vi "MS_on_off_sorting.vi"(4 "Laser gate threshold":dbl, 5 "gate_trace":waveform(dbl), 6 "Number of sweeps":i32, 7 "data_trace":waveform(dbl), 8 "IR_on_q_error_in":errorcluster, 9 "IR_on_q_in":refnum<queue>, 10 "IR_off_q_error_in":errorcluster, 11 "IR_off_q_in":refnum<queue>) -> (0 "IR_on_q_error_out":errorcluster, 1 "IR_on_q_out":refnum<queue>, 2 "IR_off_q_error_out":errorcluster, 3 "IR_off_q_out":refnum<queue>)   [LabVIEW 2020]
uses:
  <vilib>/Waveform/WDTOps.llb/WDT Number of Waveform Samples DBL.vi
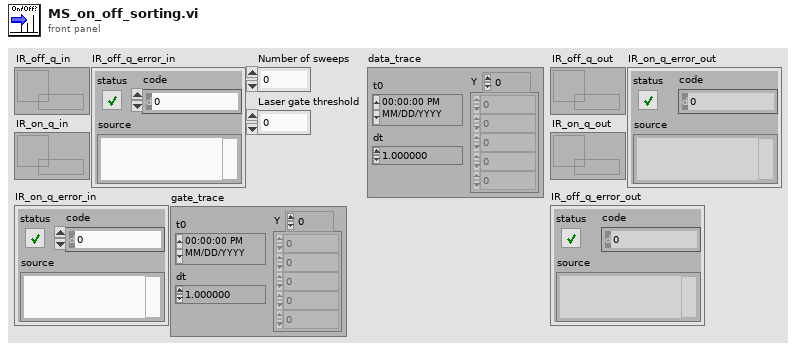
[diagram p1: front panel]
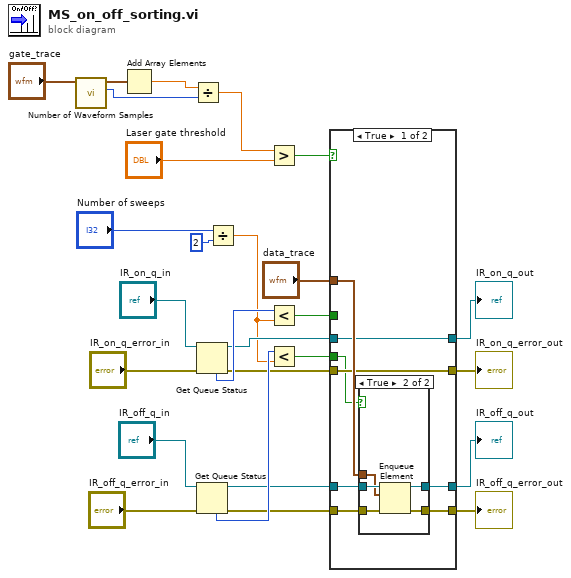
[diagram p0: block diagram]
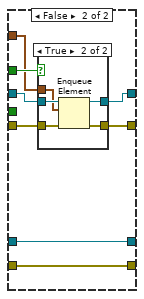
[diagram p3: hidden frame]
diagram:
  n1 = call-poly <vilib>:"Number of Waveform Samples.vi"("waveform in"="gate_trace") -> ("number of samples"=w13:i32, "waveform out"=w15:waveform(dbl))  [unwired: 8 in, 1 out]
  n2 = Add Array Elements(numeric array=w15) -> (sum=w14:dbl)
  n3 = Divide(x=w14, y=w13) -> (x/y=w18:dbl)
  n4 = Get Queue Status(queue="IR_on_q_in", error in (no error)="IR_on_q_error_in") -> (queue out=w10:refnum<queue>, error out=w9:errorcluster, # elements in queue=w20:i32)  [unwired: 1 in, 5 out]
  n5 = Get Queue Status(queue="IR_off_q_in", error in (no error)="IR_off_q_error_in") -> (queue out=w12:refnum<queue>, error out=w11:errorcluster, # elements in queue=w21:i32)  [unwired: 1 in, 5 out]
  n6 = Divide(x="Number of sweeps", y=2) -> (x/y=w2:dbl)
  n7 = Greater?(x=w18, y="Laser gate threshold") -> (0:w19:bool)
  n8 = Less?(x=w20, y=w2) -> (x < y?=w1:bool)
  n9 = Less?(x=w21, y=w2) -> (x < y?=w3:bool)
  n10 = case shown="True" w19 {
    tunnel: w12 -> [w35 w46]
    tunnel: w11 -> [w34 w45]
    tunnel: w10 -> [w30 w49]
    tunnel: w9 -> [w29 w48]
    tunnel: w1 -> [_ w50]
    tunnel: "data_trace" -> [w33 w47]
    tunnel: [w32 w46] -> w7
    tunnel: [w31 w45] -> w4
    tunnel: [w30 w44] -> w6
    tunnel: [w29 w43] -> w5
    tunnel: w3 -> [w28 _]
    frame True {
      n11 = case shown="True" w28 {
        tunnel: w35 -> [w37 w42]
        tunnel: w34 -> [w36 w41]
        tunnel: [w37 w40] -> w32
        tunnel: w33 -> [_ w39]
        tunnel: [w36 w38] -> w31
        frame False {
        }
        frame True {
          n12 = Enqueue Element(queue=w42, element=w39, error in (no error)=w41) -> (queue out=w40:refnum<queue>, error out=w38:errorcluster)  [unwired: 1 in, 1 out]
        }
      }
    }
    frame False {
      n13 = case shown="True" w50 {
        tunnel: w49 -> [w52 w57]
        tunnel: w48 -> [w51 w56]
        tunnel: [w52 w55] -> w44
        tunnel: w47 -> [_ w54]
        tunnel: [w51 w53] -> w43
        frame False {
        }
        frame True {
          n14 = Enqueue Element(queue=w57, element=w54, error in (no error)=w56) -> (queue out=w55:refnum<queue>, error out=w53:errorcluster)  [unwired: 1 in, 1 out]
        }
      }
    }
  }
  "IR_off_q_out" <- w7
  "IR_on_q_out" <- w6
  "IR_on_q_error_out" <- w5
  "IR_off_q_error_out" <- w4
